vi "IsModeAllowed.vi"(8 "error in (no error)":errorcluster, 10 "Robot Mode":string, 11 "Command in":refnum<class "Command.lvclass">) -> (0 "error out":errorcluster, 2 "Allowed Robot Mode":bool, 3 "Command out":refnum<class "Command.lvclass">)   [LabVIEW 2017, in "Command.lvclass"]
uses:
  <userlib>/836-Library/Robot/Command/Command.lvclass
  <userlib>/836-Library/Robot/Command/Command.lvclass/Command.ctl
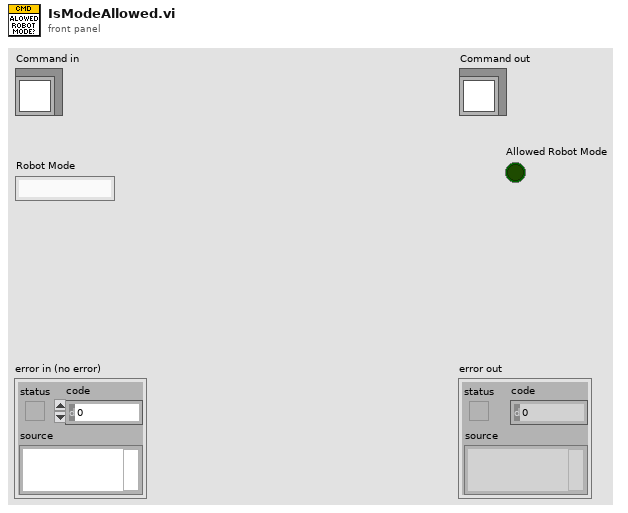
[diagram p1: front panel]
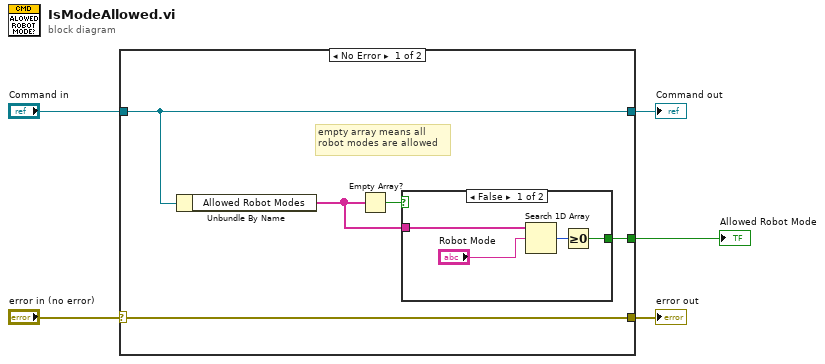
[diagram p0: block diagram]
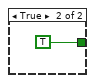
[diagram p2: hidden frame]
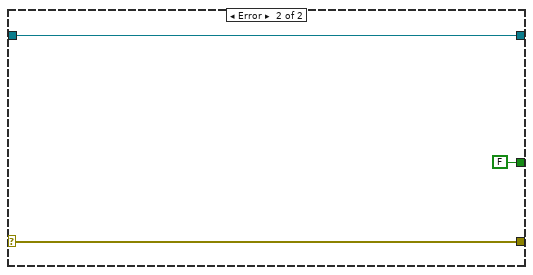
[diagram p3: hidden frame]
diagram:
  n1 = case shown="No Error" "error in (no error)" {
    selector: "error in (no error)" -> [w10 w18]
    tunnel: [w10 w18] -> w4
    tunnel: [w9 w17] -> w2
    tunnel: "Command in" -> [w9 w17]
    tunnel: [w7 FALSE] -> w1
    frame No Error {
      # "empty array means all\nrobot modes are allowed"
      n2 = Unbundle By Name(w9) -> ("Allowed Robot Modes"=w6:string[])
      n3 = Empty Array?(array=w6) -> (empty?=w8:bool)
      n4 = case shown="False" w8 {
        tunnel: [w11 TRUE] -> w7
        tunnel: w6 -> [w14 _]
        frame False {
          n5 = Search 1D Array(1D array=w14, element="Robot Mode") -> (index of element=w12:i32)  [unwired: 1 in]
          n6 = Greater Or Equal To 0?(x=w12) -> (x >= 0?=w11:bool)
        }
        frame True {
        }
      }
    }
    frame Error {
    }
  }
  "error out" <- w4
  "Command out" <- w2
  "Allowed Robot Mode" <- w1
